vi "Reset Alarm.vi"(8 "error in (no error)":errorcluster, 10 "Reset\nAlarm (T: Yes)":bool=TRUE, 11 "VISA resource name":refnum<visa-resource-name>) -> (0 "error out":errorcluster, 3 "VISA resource name out":refnum<visa-resource-name>)   [LabVIEW 2021, in "Lake Shore 336.lvlib"]
doc: "This VI resets the alarms. Alarm reset clears both the high and low status of all alarms, including latching alarms."
uses:
  <instrlib>/Lake Shore 336/Lake Shore 336.lvlib
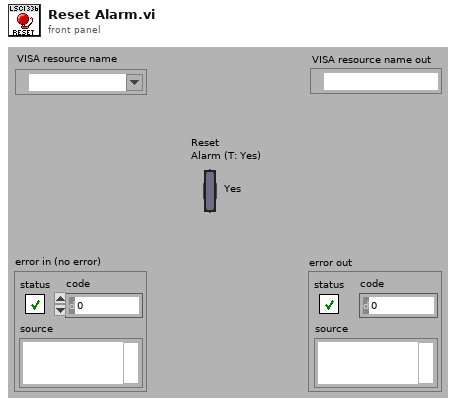
[diagram p1: front panel]
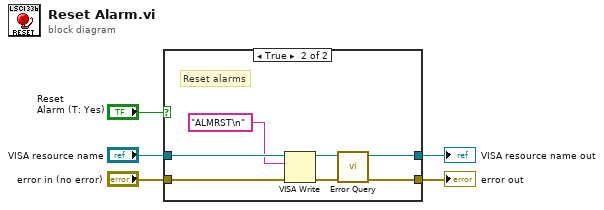
[diagram p0: block diagram]
diagram:
  n1 = case shown="True" "Reset\nAlarm (T: Yes)" {
    tunnel: "VISA resource name" -> [w7 w14]
    tunnel: "error in (no error)" -> [w6 w13]
    tunnel: [w7 w10] -> w3
    tunnel: [w6 w9] -> w2
    frame False {
      # "Do not reset alarms"
    }
    frame True {
      # "Reset alarms"
      n2 = VISA Write(VISA resource name=w14, write buffer="ALMRST\n", error in (no error)=w13) -> (VISA resource name out=w11:refnum<visa-resource-name>, error out=w12:errorcluster)  [unwired: 1 out]
      n3 = call <instrlib>:"Error Query.vi"("error in (no error)"=w12, "VISA resource name"=w11) -> ("error out"=w9:errorcluster, "VISA resource name out"=w10:refnum<visa-resource-name>)  [unwired: 7 in, 1 out]
    }
  }
  "VISA resource name out" <- w3
  "error out" <- w2
